vi "OnRestart.vi"(8 "error in (no error)":errorcluster, 11 "Game in":refnum<class "Game.lvclass">) -> (0 "error out":errorcluster, 2 "NextGame":refnum<class "Game.lvclass">, 3 "Game out":refnum<class "Game.lvclass">)   [LabVIEW 2019, in "RT_Game.lvlib" / "Game.lvclass"]
uses:
  Game.lvclass
  Game.lvclass/Game.ctl
  Read Singleplayer.vi
  Read SlideInDirection.vi
  Write Singleplayer.vi
  Write SlideInDirection.vi
  Write FlattenedNextClass.vi
  Write SwitchGame.vi
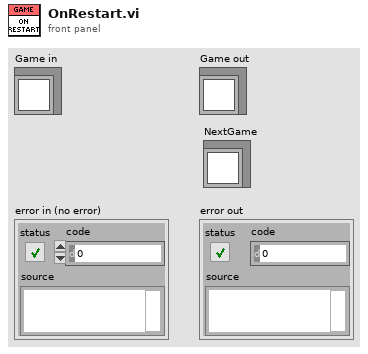
[diagram p1: front panel]
types:
  T1 = typedef "RT_Game.lvlib/Game.lvclass/ScreenSide.ctl" = enum16{"up", "down", "left", "right", "none"}
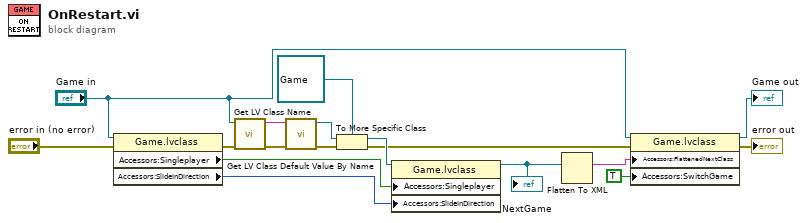
[diagram p0: block diagram]
diagram:
  n1 = property class="Game.lvclass"(reference="Game in", error in="error in (no error)") -> (error out=w4:errorcluster, "Accessors:Singleplayer"=w3:bool, "Accessors:SlideInDirection"=w2:T1)  [unwired: 1 out]
  n2 = call <vilib>:"Get LV Class Name.vi"("error in (no error)"=w4, "object"="Game in") -> ("error out"=w11:errorcluster, "class name"=w12:string)  [unwired: 8 in]
  n3 = call <vilib>:"Get LV Class Default Value By Name.vi"("error in (no error)"=w11, "class name"=w12) -> ("error out"=w10:errorcluster, "object"=w14:refnum<class>)  [unwired: 8 in]
  n4 = To More Specific Class(target class=refnum<class "Game.lvclass"> refnum ("Game out"), reference=w14, error in=w10) -> (specific class reference=w15:refnum<class "Game.lvclass">, error out=w13:errorcluster)
  n5 = property class="Game.lvclass"(reference=w15, "Accessors:Singleplayer"=w3, "Accessors:SlideInDirection"=w2) -> (reference out=w6:refnum<class "Game.lvclass">)  [unwired: 1 in, 1 out]
  "NextGame" <- w6
  n6 = Flatten To XML(anything=w6) -> (xml string=w5:string)
  n7 = property class="Game.lvclass"(reference="Game in", error in=w13, "Accessors:FlattenedNextClass"=w5, "Accessors:SwitchGame"=TRUE ("SwitchGame")) -> (reference out=→"Game out":refnum<class "Game.lvclass">, error out=→"error out":errorcluster)
